vi "CRITPdll.vi"(8 "error in (no error)":errorcluster, 11 "z":dbl[](array[numeric])) -> (0 "error out":errorcluster, 3 "Outputs":T1)   [LabVIEW 2016]
doc: "subroutine CRITPdll(z, tc, pc, dc, ierr, herr, herr_length)\n\nCalculate critical parameters as a function of composition.\n\nINPUTS:\nz -- Composition (array of mole fractions)\n\nOUTPUTS:\ntc -- Critical temperature [K]\npc -- Critical pressure [kPa]\ndc -- Critical density [mol/L]\nierr -- Error flag: See subroutine CRTHMX for error numbers\nherr -- Error string (character*255)\nherr_length -- length of variable herr (default: 255)"
uses:
  REFPROP.DLL
panel:
  # "REFPROP-CRITPdll.vi"
  # "void  CRITPdll(double *z, double *tc, double *pc, double *dc, int32_t *ierr, CStr herr, int32_t herr_length)"
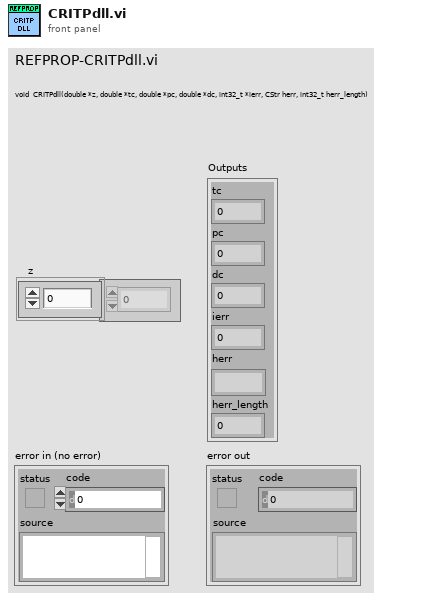
[diagram p1: front panel]
types:
  T1 = cluster{"tc":dbl, "pc":dbl, "dc":dbl, "ierr":i32, "herr":string, "herr_length":i32}
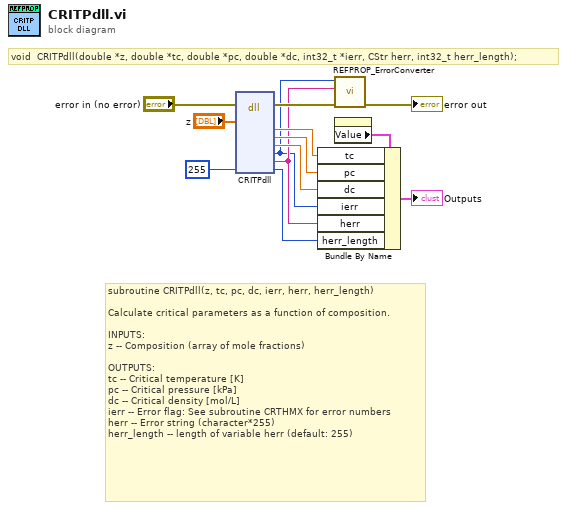
[diagram p0: block diagram]
diagram:
  # "void  CRITPdll(double *z, double *tc, double *pc, double *dc, int32_t *ierr, CStr herr, int32_t herr_length);"
  # "subroutine CRITPdll(z, tc, pc, dc, ierr, herr, herr_length)\n\nCalculate critical parameters as a function of composition.\n\nINPUTS:\nz -- Composition (array of mole fractions)\n\nOUTPUTS:\ntc -- Critical temperature [K]\npc -- Critical pressure [kPa]\ndc -- Critical density [mol/L]\nierr -- Error flag: See subroutine CRTHMX for error numbers\nherr -- Error string (character*255)\nherr_length -- length of variable herr (default: 255)"
  n1 = dll-call lib="S:/009 - Testing/02 - Performance Testing/REFPROP/REFPROP.*" fn="CRITPdll"(error in="error in (no error)", "z"="z", "herr_length"=255 ("ln")) -> (error out=w11:errorcluster, "tc"=w3:dbl, "pc"=w4:dbl, "dc"=w5:dbl, "ierr"=w1:i32, "herr"=w2:string, "herr_length"=w6:i32)  [unwired: 9 in, 1 out]
  n2 = call "REFPROP_ErrorConverter.vi"("error in (no error)"=w11, "Error Message"=w2, "Error Code"=w1) -> ("error out"=→"error out":errorcluster)  [unwired: 8 in]
  n3 = property on="Outputs" class="Clust (strict)"() -> ("Value"=w8:T1)  [unwired: 2 in, 2 out]
  n4 = Bundle By Name(cluster=w8, "tc"=w3, "pc"=w4, "dc"=w5, "ierr"=w1, "herr"=w2, "herr_length"=w6) -> (→"Outputs":T1)
